vi "Determine Warning - efficient but not scalable.vi"(6 "강풍":dbl, 7 "현재 풍속":dbl, 8 "에러 입력(에러 없음)":errorcluster, 9 "최저 온도":dbl, 10 "최고 온도":dbl, 11 "현재 온도":dbl) -> (0 "경고 출력":errorcluster caption="에러 출력", 1 "경고?":bool, 2 "경고 텍스트":string)   [LabVIEW 2010]
doc: "이 VI는 LabVIEW Core II 과정의 연습문제에 대한 해답입니다. 이 연습문제에서 상속된 코드를 가지고 읽기 쉽고 관리하기 쉽도록 개선하게 됩니다."
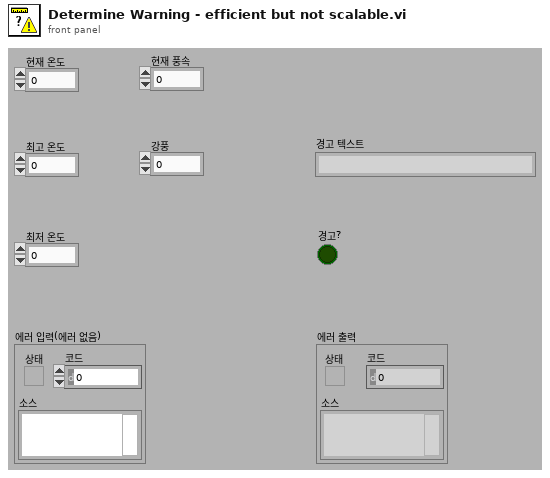
[diagram p1: front panel]
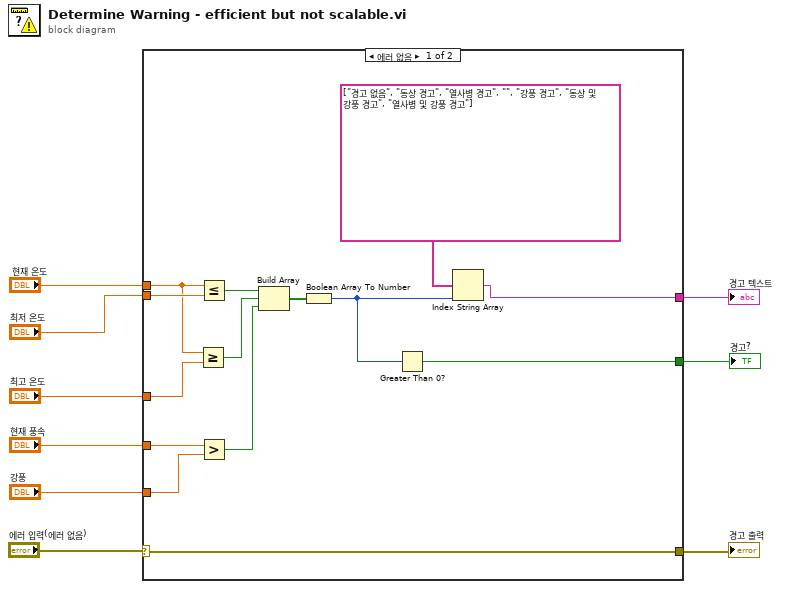
[diagram p0: block diagram]
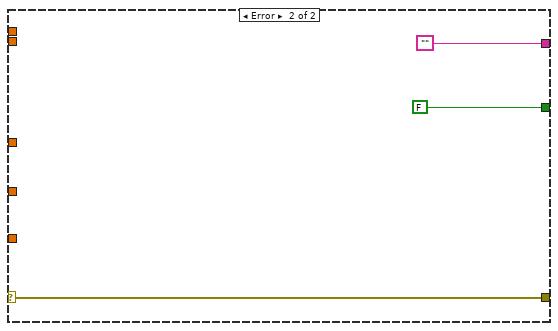
[diagram p2: hidden frame]
diagram:
  n1 = case shown="에러 없음" "에러 입력(에러 없음)" {
    selector: "에러 입력(에러 없음)" -> [w11 w26]
    tunnel: "최고 온도" -> [w23 _]
    tunnel: "최저 온도" -> [w22 _]
    tunnel: "현재 풍속" -> [w21 _]
    tunnel: "강풍" -> [w20 _]
    tunnel: "현재 온도" -> [w19 _]
    tunnel: [w13 ""] -> w4
    tunnel: [w12 FALSE] -> w3
    tunnel: [w11 w26] -> w1
    frame No Error {
      n2 = Greater Or Equal?(x=w19, y=w23) -> (x >= y?=w17:bool)
      n3 = Less Or Equal?(x=w19, y=w22) -> (x <= y?=w18:bool)
      n4 = Greater?(x=w21, y=w20) -> (0:w15:bool)
      n5 = Build Array(w18, w17, w15) -> (w16:bool[])
      n6 = Boolean Array To Number(Boolean array=w16) -> (number=w10:u32)
      n7 = Greater Than 0?(x=w10) -> (x > 0?=w12:bool)
      n8 = Index String Array(1:w10, 2:string[] ["경고 없음", "동상 경고", "열사병 경고", "", "강풍 경고", "동상 및 강풍 경고", "열사병 및 강풍 경고"]) -> (0:w13:string)  [unwired: 1 out]
    }
    frame Error {
    }
  }
  "경고 출력" <- w1
  "경고 텍스트" <- w4
  "경고?" <- w3
